vi "Extract subclasses from Flow device.vi"(9 "Data In":string, 10 "Class":string, 11 "Heater Device Settings in":T1) -> (1 "Data out":string, 3 "Heater Device Settings out":T1)   [LabVIEW 2016, in "Mercury iXX.lvlib" / "Flow.lvlib"]
uses:
  Flow.lvlib
  Controls/Flow Device (Read).ctl
  Controls/Manufacturing Data.ctl
  Controls/Flow Signals Cluster.ctl
  Mercury iXX.lvlib
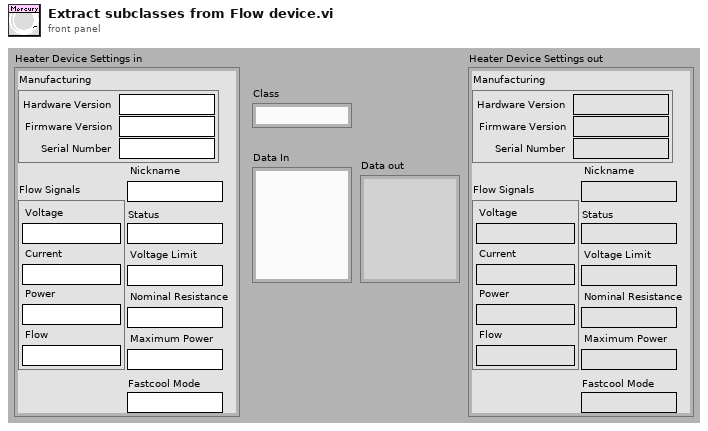
[diagram p1: front panel]
types:
  T1 = typedef "Mercury iXX.lvlib/Flow.lvlib/Flow Device (Read).ctl" = cluster{"Manufacturing":T2, "Nickname":string, "Voltage Limit":string, "Nominal Resistance":string, "Maximum Power":string, "Flow Signals":T3, "Status":string, "Fastcool Mode":string}
  T2 = typedef "Mercury iXX.lvlib/Manufacturing Data.ctl" = cluster{"Hardware Version":string, "Firmware Version":string, "Serial Number":string}
  T3 = typedef "Mercury iXX.lvlib/Flow.lvlib/Flow Signals Cluster.ctl" = cluster{"Voltage":string, "Current":string, "Power":string, "Flow":string}
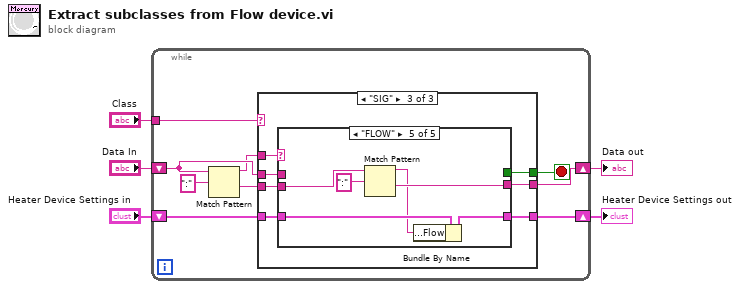
[diagram p0: block diagram]
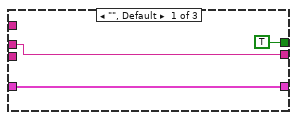
[diagram p2: hidden frame]
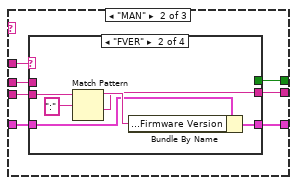
[diagram p3: hidden frame]
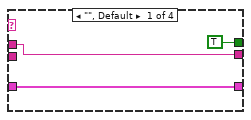
[diagram p4: hidden frame]
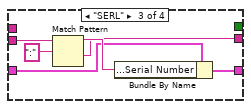
[diagram p5: hidden frame]
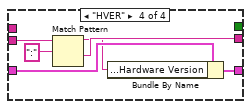
[diagram p6: hidden frame]
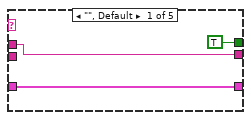
[diagram p7: hidden frame]
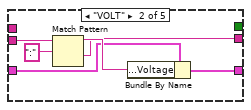
[diagram p8: hidden frame]
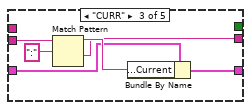
[diagram p9: hidden frame]
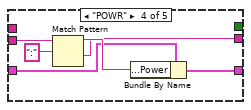
[diagram p10: hidden frame]
diagram:
  n1 = while {
    tunnel: "Class" -> [w9]
    shift-right: [w10] -> w4
    shift-left: "Data In" -> [w7]
    shift-right: [w12] -> w3
    shift-left: "Heater Device Settings in" -> [w13]
    stop <- w8 stop-if-true
    n2 = Match Pattern(string=w7, regular expression=":") -> (before substring=w6:string, after substring=w11:string)  [unwired: 3 out]
    n3 = case shown="\"SIG\"" w9 {
      tunnel: w13 -> [w17 w24 w52]
      tunnel: [w17 w23 w51] -> w12
      tunnel: w11 -> [_ w22 w50]
      tunnel: [w15 w21 w49] -> w10
      tunnel: [TRUE w19 w47] -> w8
      tunnel: w7 -> [w15 w18 w46]
      tunnel: w6 -> [_ w20 w48]
      frame "", Default {
      }
      frame "MAN" {
        n4 = case shown="\"FVER\"" w20 {
          tunnel: w24 -> [w26 w30 w36 w45]
          tunnel: [w26 w29 w35 w44] -> w23
          tunnel: w22 -> [_ w31 w37 w43]
          tunnel: [w25 w28 w34 w42] -> w21
          tunnel: [TRUE _ _ _] -> w19
          tunnel: w18 -> [w25 _ _ _]
          frame "", Default {
          }
          frame "FVER" {
            n5 = Match Pattern(string=w31, regular expression=":") -> (before substring=w32:string, after substring=w28:string)  [unwired: 3 out]
            n6 = Bundle By Name(cluster=w30, "Manufacturing.Firmware Version"=w32) -> (w29:T1)
          }
          frame "SERL" {
            n7 = Match Pattern(string=w37, regular expression=":") -> (before substring=w38:string, after substring=w34:string)  [unwired: 3 out]
            n8 = Bundle By Name(cluster=w36, "Manufacturing.Serial Number"=w38) -> (w35:T1)
          }
          frame "HVER" {
            n9 = Match Pattern(string=w43, regular expression=":") -> (before substring=w40:string, after substring=w42:string)  [unwired: 3 out]
            n10 = Bundle By Name(cluster=w45, "Manufacturing.Hardware Version"=w40) -> (w44:T1)
          }
        }
      }
      frame "SIG" {
        n11 = case shown="\"FLOW\"" w48 {
          tunnel: w52 -> [w53 w58 w64 w70 w78]
          tunnel: [w53 w59 w63 w71 w75] -> w51
          tunnel: w50 -> [_ w57 w65 w69 w77]
          tunnel: [w54 w56 w62 w68 w76] -> w49
          tunnel: [TRUE _ _ _ _] -> w47
          tunnel: w46 -> [w54 _ _ _ _]
          frame "", Default {
          }
          frame "VOLT" {
            n12 = Match Pattern(string=w57, regular expression=":") -> (before substring=w60:string, after substring=w56:string)  [unwired: 3 out]
            n13 = Bundle By Name(cluster=w58, "Flow Signals.Voltage"=w60) -> (w59:T1)
          }
          frame "CURR" {
            n14 = Match Pattern(string=w65, regular expression=":") -> (before substring=w66:string, after substring=w62:string)  [unwired: 3 out]
            n15 = Bundle By Name(cluster=w64, "Flow Signals.Current"=w66) -> (w63:T1)
          }
          frame "POWR" {
            n16 = Match Pattern(string=w69, regular expression=":") -> (before substring=w72:string, after substring=w68:string)  [unwired: 3 out]
            n17 = Bundle By Name(cluster=w70, "Flow Signals.Power"=w72) -> (w71:T1)
          }
          frame "FLOW" {
            n18 = Match Pattern(string=w77, regular expression=":") -> (before substring=w74:string, after substring=w76:string)  [unwired: 3 out]
            n19 = Bundle By Name(cluster=w78, "Flow Signals.Flow"=w74) -> (w75:T1)
          }
        }
      }
    }
  }
  "Data out" <- w4
  "Heater Device Settings out" <- w3
